vi "3_AdvancedDemo_MHT3.vi"() -> ()   [LabVIEW 2020]
uses:
  Types/MH_UIThread_Cmds.ctl
  _lib/PQ/MultiHarp/MH_InitInfo.ctl
  Types/MH_UIThread_Data.ctl
  Types/MH_InputChannel.ctl
  _lib/PQ/MultiHarp/MH_RefSource.ctl
  _lib/PQ/MultiHarp/mhlib_x86_x64_UIThread.llb/MH_DllPath_global.vi
  <vilib>/Utility/error.llb/DialogType.ctl
  <vilib>/ErrorRing/Error Ring.xnode
  <vilib>/Utility/error.llb/Error Cluster From Error Code.vi
  Types/MH_DataProcThread_QCmds.ctl
  Types/MH_DataProcThread_QData.ctl
  Types/MH_VisThread_QCmds.ctl
  Types/MH_VisThread_QData.ctl
  Types/MH_VisThread_Data.ctl
  _lib/PQ/MultiHarp/MH_LibVersion_global.vi
  _lib/PQ/MultiHarp/MH_MeasMode.ctl
  Types/MH_SetInpChanData.ctl
  Types/MH_SetInpChanCmds.ctl
panel:
  in  "Settings":bool=TRUE
  in  "Run continuously":bool caption="Conti."
  in  "Start":bool
  in  "Scale":bool
  out "CountRates":i32[](graph)
  in  "AllChannels":T1={"Enable"=TRUE, "Offset"=0, "Level"=-100, "Edge"=0, "DeadTime"=1000, "UseDeadTime"=FALSE, "SetEnableAllChan"=TRUE, "SetEdgeAllChan"=TRUE, "SetLevelAllChan"=TRUE, "SetOffsetAllChan"=TRUE, "SetUseDTAllChan"=TRUE, "SetDeadTAllChan"=TRUE} {"DeadTime" min=800 max=160000 step=1; "Edge" items=["falling", "rising"]; "Offset" min=-100000 max=100000 step=10; "Level" min=-1200 max=1200 step=1}
  in  "HistoAcqTime":dbl=1.0 caption="Hist.Int.Time  s" min=0.1 max=360000.0 step=0.1
  in  "AcqTime":i32=360000000 caption="T3Acqu.       ms" min=1 max=360000 step=1
  in  "Binning":i32(ring) caption="Resol.            ps" items=["10", "20", "40", "80", "160", "320", "640", "1280", "2560", "5120", "10240", "20480", "40960", "81920", "163840", "327680", "655360", "1310720", "2621440", "5242880", "10485760", "20971520", "41943040"]
  in  "HistoOffset":i32 caption="Offset            ns" min=0 max=100000000 step=1
  out "DeltaT":dbl=6.553665536655367 caption="T.Tr.Resol.   ms" format="%.2f"
  in  "BitShift":i32=15 min=0 max=32 step=1
  in  "OvlLevel":u32=4294967295 caption="Ovl.Level" min=1024 max=65536 step=1024
  in  "StopOvl.":bool=TRUE
  out "TTraceGraph":T2(graph)={49.38852226226715, "Resolution"=0.00655367864414373, "Histogram"=[]}
  out "HistoGraph":cluster{dbl, "Resol":dbl, "Histos":u32[][]}(graph)={0.0, "Resol"=0.08, "Histos"=[]}
  in  "SyncDeadTime":i32=1000 caption="Dead T.   ps" min=800 max=160000 step=1
  in  "UseDeadTime":bool caption="Use DT."
  in  "SyncEdge":i32(ring) caption="Edge" items=["falling", "rising"]
  in  "SyncDivider":i32(ring) caption="Divider" items=["1", "2", "4", "8", "16"]
  in  "SyncOffset":i32 caption="Offset      ps" min=-100000 max=100000 step=10
  in  "SyncLevel":i32=-100 caption="Level      mV" min=-1200 max=1200 step=1
  in  "Channels":T3[](array[typedef])=[{"Name"="Inp.Chan 1", "Enable"=TRUE, "Edge"=0, "Level"=-100, "Offset"=0, "UseDeadTime"=FALSE, "DeadTime"=1000}, {"Name"="Inp.Chan 2", "Enable"=TRUE, "Edge"=0, "Level"=-100, "Offset"=0, "UseDeadTime"=FALSE, "DeadTime"=1000}, {"Name"="Inp.Chan 3", "Enable"=TRUE, "Edge"=0, "Level"=-100, "Offset"=0, "UseDeadTime"=FALSE, "DeadTime"=1000}, {"Name"="Inp.Chan 4", "Enable"=TRUE, "Edge"=0, "Level"=-100, "Offset"=0, "UseDeadTime"=FALSE, "DeadTime"=1000}, {"Name"="Inp.Chan 5", "Enable"=TRUE, "Edge"=0, "Level"=-100, "Offset"=0, "UseDeadTime"=FALSE, "DeadTime"=1000}, {"Name"="Inp.Chan 6", "Enable"=TRUE, "Edge"=0, "Level"=-100, "Offset"=0, "UseDeadTime"=FALSE, "DeadTime"=1000}, {"Name"="Inp.Chan 7", "Enable"=TRUE, "Edge"=0, "Level"=-100, "Offset"=0, "UseDeadTime"=FALSE, "DeadTime"=1000}, {"Name"="Inp.Chan 8", "Enable"=TRUE, "Edge"=0, "Level"=-100, "Offset"=0, "UseDeadTime"=FALSE, "DeadTime"=1000}, {"Name"="Inp.Chan 9", "Enable"=TRUE, "Edge"=0, "Level"=-100, "Offset"=0, "UseDeadTime"=FALSE, "DeadTime"=1000}, {"Name"="Inp.Chan 10", "Enable"=TRUE, "Edge"=0, "Level"=-100, "Offset"=0, "UseDeadTime"=FALSE, "DeadTime"=1000}, {"Name"="Inp.Chan 11", "Enable"=TRUE, "Edge"=0, "Level"=-100, "Offset"=0, "UseDeadTime"=FALSE, "DeadTime"=1000}, {"Name"="Inp.Chan 12", "Enable"=TRUE, "Edge"=0, "Level"=-100, "Offset"=0, "UseDeadTime"=FALSE, "DeadTime"=1000}, {"Name"="Inp.Chan 13", "Enable"=TRUE, "Edge"=0, "Level"=-100, "Offset"=0, "UseDeadTime"=FALSE, "DeadTime"=1000}, {"Name"="Inp.Chan 14", "Enable"=TRUE, "Edge"=0, "Level"=-100, "Offset"=0, "UseDeadTime"=FALSE, "DeadTime"=1000}, {"Name"="Inp.Chan 15", "Enable"=TRUE, "Edge"=0, "Level"=-100, "Offset"=0, "UseDeadTime"=FALSE, "DeadTime"=1000}, {"Name"="Inp.Chan 16", "Enable"=TRUE, "Edge"=0, "Level"=-100, "Offset"=0, "UseDeadTime"=FALSE, "DeadTime"=1000}] {"DeadTime" min=800 max=160000 step=1; "Edge" items=["falling", "rising"]; "Offset" min=-100000 max=100000 step=10; "Level" min=-1200 max=1200 step=1}
  out "SyncRate":string="Sync Rate: 4999940 cps\n"
  out "OverRun":bool caption="Overrun:"
  out "Status":string="Elements in Q: 0"
  # "All Channels"
  # "Acquisition"
  # "Sync"
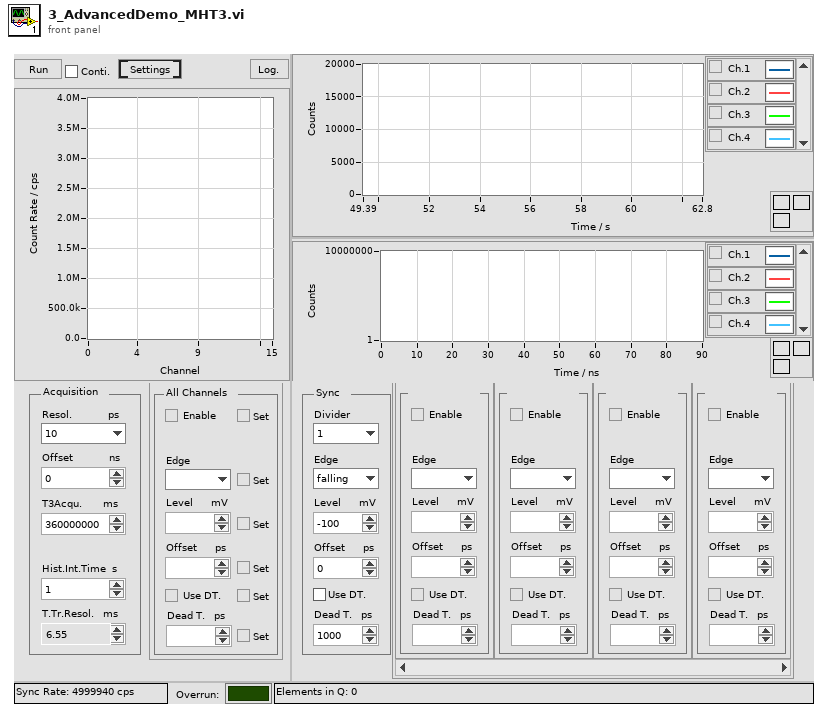
[diagram p1: front panel]
types:
  T1 = cluster{"Enable":bool, "Offset":i32, "Level":i32, "Edge":i32, "DeadTime":i32, "UseDeadTime":bool, "SetEnableAllChan":bool, "SetEdgeAllChan":bool, "SetLevelAllChan":bool, "SetOffsetAllChan":bool, "SetUseDTAllChan":bool, "SetDeadTAllChan":bool}
  T2 = cluster{dbl, "Resolution":dbl, "Histogram":u32[][]}
  T3 = typedef "MH_InputChannel.ctl" = cluster{"Name":string, "Enable":bool, "Edge":i32, "Level":i32, "Offset":i32, "UseDeadTime":bool, "DeadTime":i32}
  T4 = typedef "MH_DataProcThread_QCmds.ctl" = enum16{"Exit", "Proc", "Init", "SetShift", "SetNumChannels", "SetHistAcqTime"}
  T5 = typedef "MH_VisThread_Data.ctl" = cluster{"Resol":dbl, "DeltaT":dbl, "NumChannels":i32}
  T6 = typedef "MH_VisThread_QData.ctl" = cluster{"Histos":u32[][], "Cmd":T7, "TimeTrace":u32[][], "Bin":i32, "Total bin":u64, "Status":string, "Resol":dbl, "DeltaT":dbl, "nChannels":i32}
  T7 = typedef "MH_VisThread_QCmds.ctl" = enum16{"_none_", "Resol", "nChannels", "DeltaT", "Histo", "TTrace", "Status"}
  T8 = typedef "MH_DataProcThread_QData.ctl" = cluster{"Cmd":T4, "nActual":i32, "Buffer":u32[], "TickCount":u32, "Param":i32}
  T9 = typedef "MH_UIThread_Data.ctl" = cluster{"Init Info":T10, "DevIdx":i32, "SyncDivider":i32, "SyncOffset":i32, "SyncLevel":i32, "Channels":T3[], "CurrentChannels":i32[], "AcqTime":i32, "Binning":i32, "HistoOffset":i32, "HistoLen":i32, "StopOvl.":bool, "OvlLevel":u32, "SyncEdge":i32, "StartMeas":bool, "HistoLength":i32, "Resolution":dbl, "Run cont.":bool, "Status":string, "SyncRate":i32, "BitShift":i32, "HistoAcqTime":dbl, "SyncRateStart":i32, "UseDeadTime":bool, "SyncDeadTime":i32, "SetInpChan":T11[]}
  T10 = typedef "MH_InitInfo.ctl" = cluster{"Library Version":string, "Serial No.":string, "Model":string, "Partnum":string, "Version":string, "features":i32, "nchannels":i32, "Base Resolution":dbl, "Bin Steps":i32}
  T11 = typedef "MH_SetInpChanData.ctl" = cluster{"Channel":i32, "Cmds":T12[], "Changed":cluster{"Name":bool, "Enable":bool, "Edge":bool, "Level":bool, "Offset":bool, "UseDeadTime":bool, "DeadTime":bool}}
  T12 = typedef "MH_SetInpChanCmds.ctl" = enum16{"SetInpChanEnable", "SetInpChanOffset", "SetInpChanDeadTime", "SetInpChanTrg"}
  T13 = typedef "MH_UIThread_Cmds.ctl" = enum16{"Idle", "Init", "SetInpChan", "SetSyncDivider", "SetSyncTrg", "SetSyncOffset", "SetSyncDeadTime", "SetBinning", "SetHistoOffset", "SetHistoLen", "SetStopOvl", "SetBitShift", "SetHistoAcqTime", "GetRates", "GetAllRates", "StartMeas", "StopMeas", "AbortMeas", "GetResolution", "GetHistos", "GetAllHistos", "ReadFiFo", "WriteStatus", "Resize", "EnableControls", "DisableControls", "Error", "Exit"}
  T14 = enum8{"Enabled", "Disabled", "Disabled and Grayed Out"}
  T15 = cluster{"[0]":bool, "[1]":bool, "[2]":bool, "[3]":bool, "[4]":bool, "[5]":bool}
  T16 = typedef "MH_MeasMode.ctl" = i32
  T17 = typedef "MH_RefSource.ctl" = enum16{"INTERNAL", "EXTERNAL_10MHZ", "WR_MASTER_GENERIC", "WR_SLAVE_GENERIC", "WR_GRANDM_GENERIC", "EXTN_GPS_PPS", "EXTN_GPS_PPS_UART", "WR_MASTER_MHARP", "WR_SLAVE_MHARP", "WR_GRANDM_MHARP"}
  T18 = typedef "DialogType.ctl" = u16
  T19 = cluster{"T0":dbl, "dt":dbl, "TimeTrace_out":u32[][]}
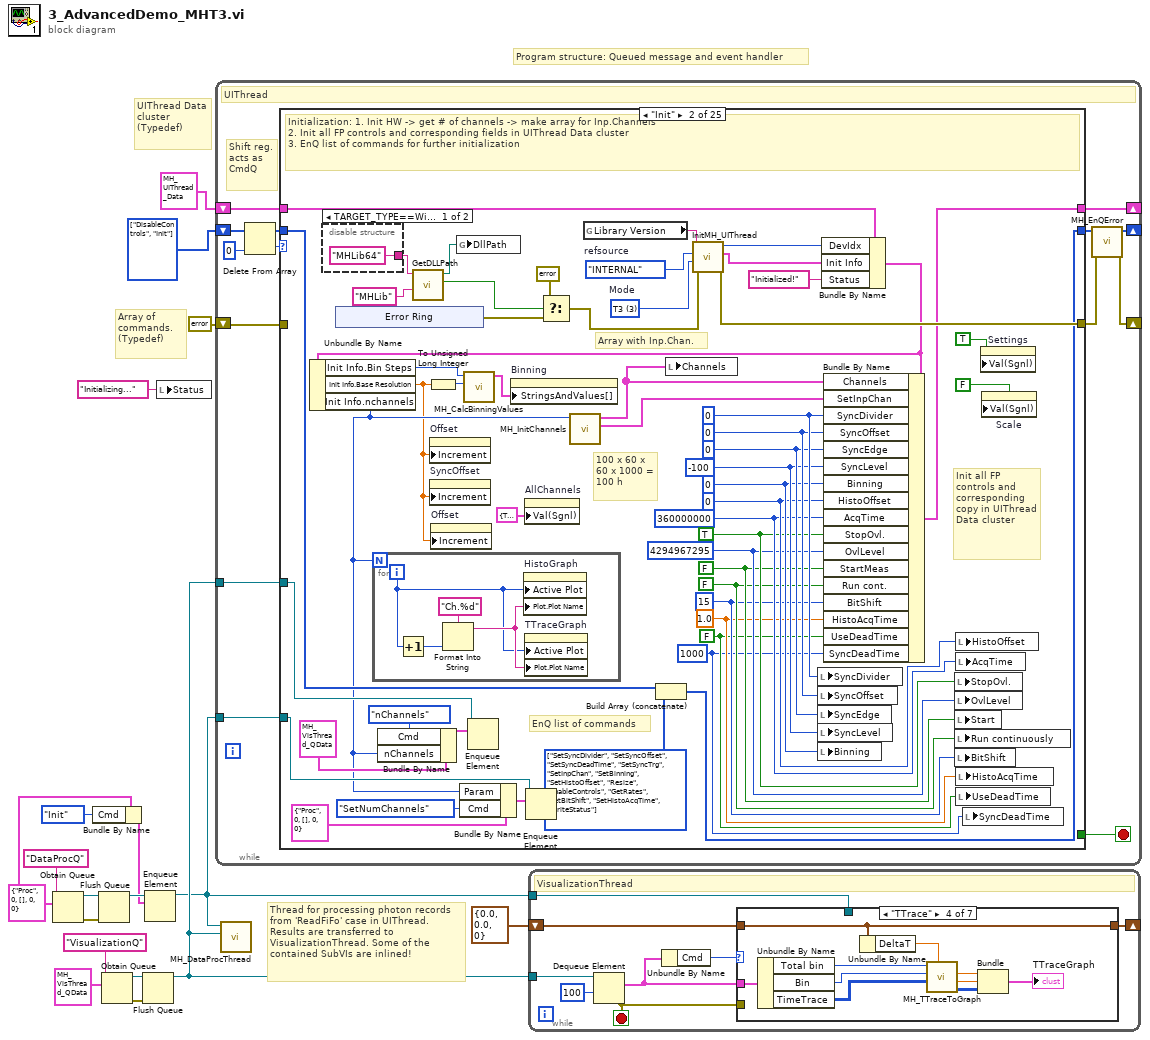
[diagram p0: block diagram]
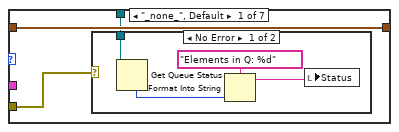
[diagram p2: hidden frame]
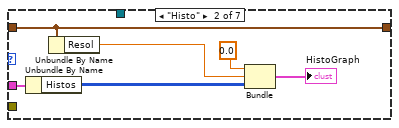
[diagram p4: hidden frame]
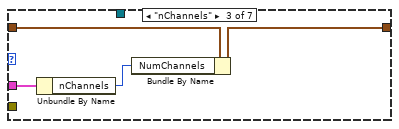
[diagram p5: hidden frame]
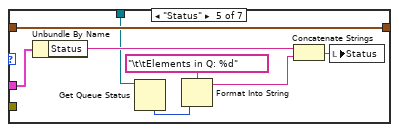
[diagram p6: hidden frame]
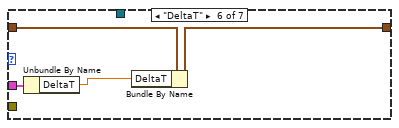
[diagram p7: hidden frame]
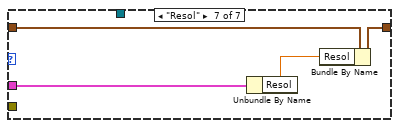
[diagram p8: hidden frame]
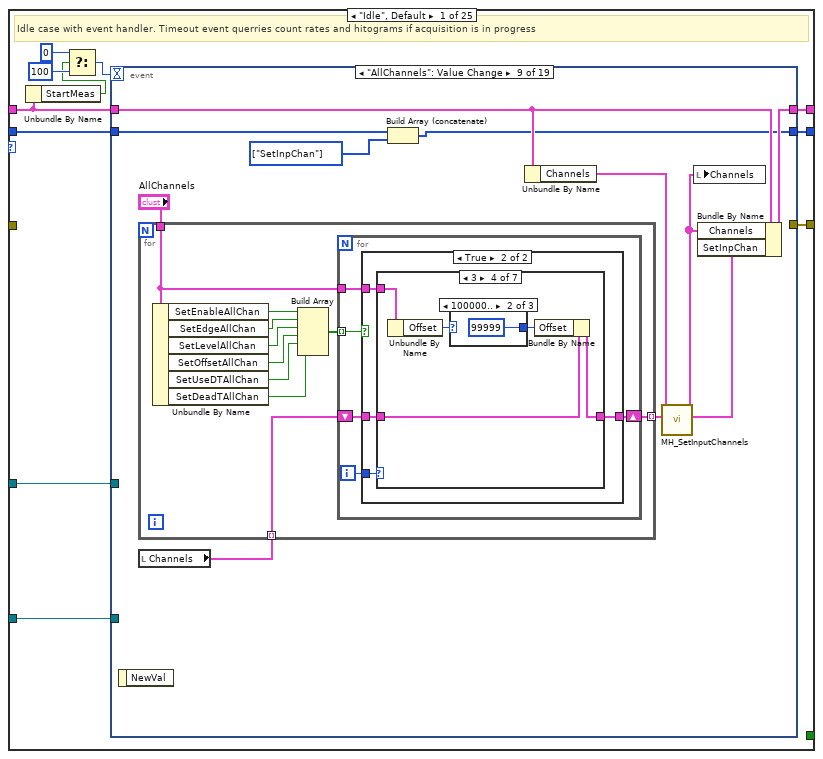
[diagram p9: hidden frame]
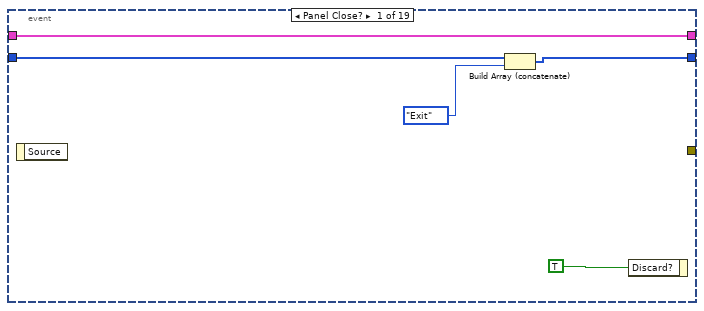
[diagram p10: hidden frame]
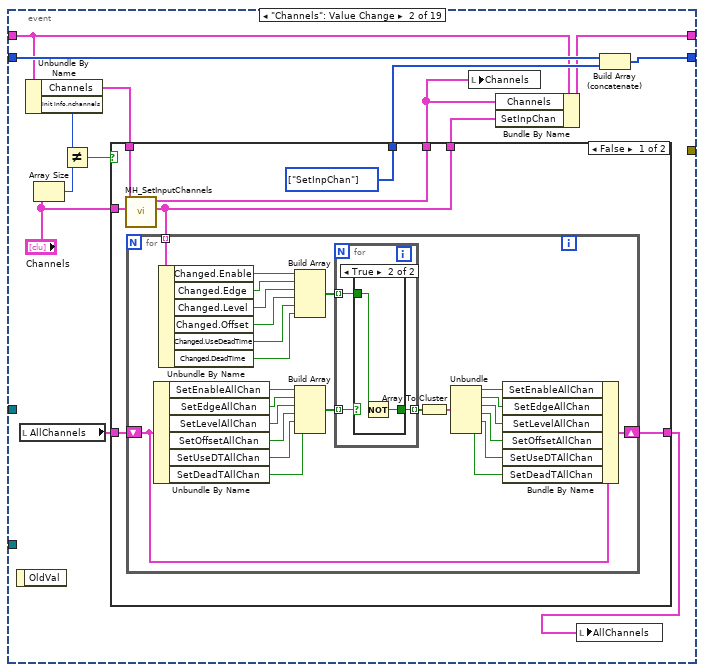
[diagram p11: hidden frame]
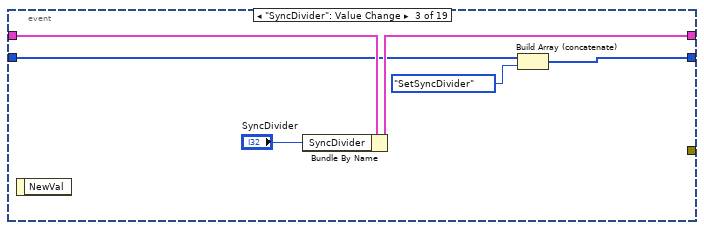
[diagram p14: hidden frame]
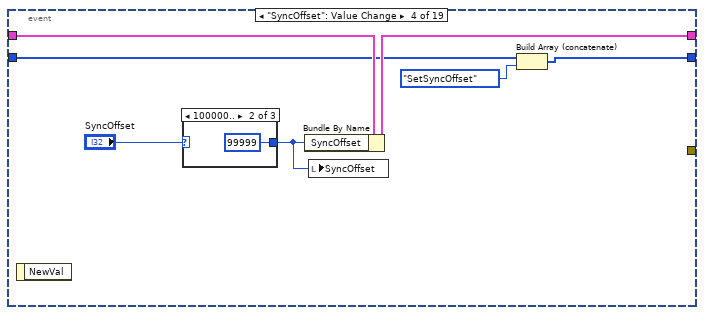
[diagram p15: hidden frame]
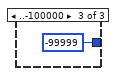
[diagram p17: hidden frame]
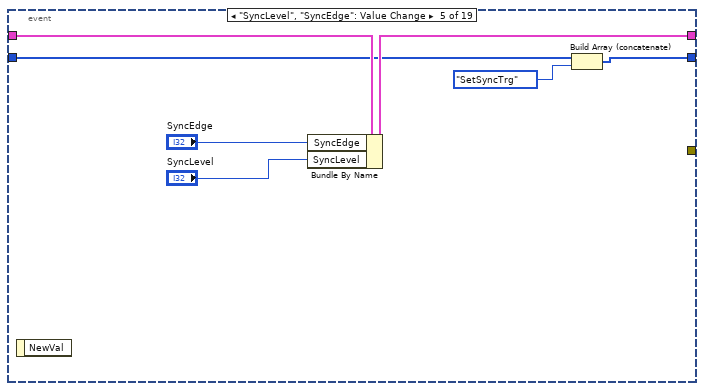
[diagram p18: hidden frame]
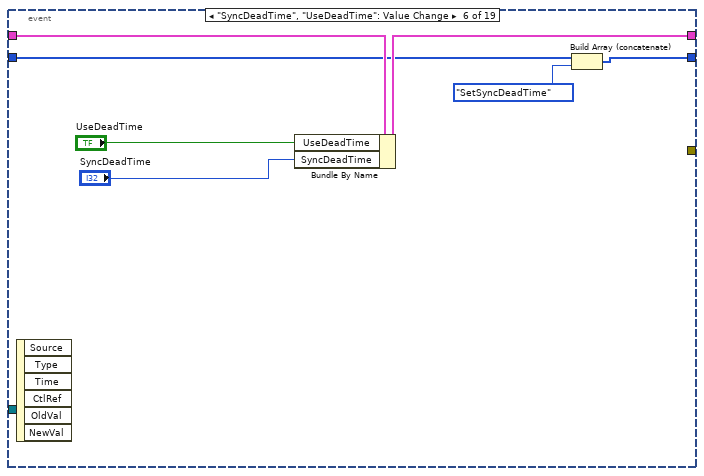
[diagram p19: hidden frame]
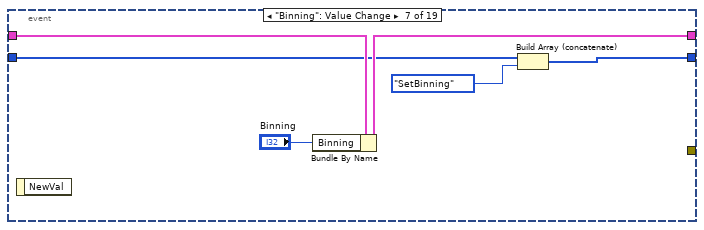
[diagram p20: hidden frame]
diagram:
  w4 = T8 {"Cmd"=enum."Proc", "nActual"=0, "Buffer"=[], "TickCount"=0, "Param"=0} ("MH_DataProcThread_QData")
  w17 = T13[] [enum."DisableControls", enum."Init"] items=["Idle", "Init", "SetInpChan", "SetSyncDivider", "SetSyncTrg", "SetSyncOffset", "SetSyncDeadTime", "SetBinning", "SetHistoOffset", "SetHistoLen", "SetStopOvl", "SetBitShift", "SetHistoAcqTime", "GetRates", "GetAllRates", "StartMeas", "StopMeas", "AbortMeas", "GetResolution", "GetHistos", "GetAllHistos", "ReadFiFo", "WriteStatus", "Resize", "EnableControls", "DisableControls", "Error", "Exit"]
  # "Thread for processing photon records from 'ReadFiFo' case in UIThread. Results are transferred to VisualizationThread. Some of the contained SubVIs are inlined!"
  # "Array of commands.\n(Typedef)"
  # "Program structure: Queued message and event handler"
  # "UIThread Data cluster\n(Typedef)"
  n1 = Obtain Queue(name (unnamed)="DataProcQ", element data type=w4) -> (queue out=w14:refnum<queue>, error out=w13:errorcluster)  [unwired: 3 in, 1 out]
  n2 = Bundle By Name(cluster=w4, "Cmd"=MH_DataProcThread_QCmds."Init") -> (w2:T8)
  n3 = Flush Queue(queue=w14, error in (no error)=w13) -> (queue out=w5:refnum<queue>)  [unwired: 2 out]
  n4 = Obtain Queue(name (unnamed)="VisualizationQ", element data type=T6 {"Histos"=[], "Cmd"=enum."_none_", "TimeTrace"=[], "Bin"=0, "Total bin"=0, "Status"="", "Resol"=0.0, "DeltaT"=0.0, "nChannels"=0} ("MH_GUIThread_QData")) -> (queue out=w12:refnum<queue>, error out=w11:errorcluster)  [unwired: 3 in, 1 out]
  n5 = Flush Queue(queue=w12, error in (no error)=w11) -> (queue out=w7:refnum<queue>)  [unwired: 2 out]
  n6 = Enqueue Element(queue=w5, element=w2) -> (queue out=w1:refnum<queue>)  [unwired: 2 in, 2 out]
  n7 = local write "Status"("Initializing..." ("Status")) -> ()
  n8 = while {
    shift-right: [w21] -> _
    shift-left: w17 -> [w28]
    shift-right: [w31] -> _
    shift-left: T9 {"Init Info"={"Library Version"="", "Serial No."="", "Model"="", "Partnum"="", "Version"="", "features"=0, "nchannels"=0, "Base Resolution"=0.0, "Bin Steps"=0}, "DevIdx"=0, "SyncDivider"=1, "SyncOffset"=0, "SyncLevel"=50, "Channels"=[], "CurrentChannels"=[], "AcqTime"=1, "Binning"=1, "HistoOffset"=1, "HistoLen"=1024, "StopOvl."=FALSE, "OvlLevel"=1024, "SyncEdge"=10, "StartMeas"=FALSE, "HistoLength"=0, "Resolution"=0.0, "Run cont."=FALSE, "Status"="", "SyncRate"=0, "BitShift"=0, "HistoAcqTime"=0.0, "SyncRateStart"=0, "UseDeadTime"=FALSE, "SyncDeadTime"=800, "SetInpChan"=[]} -> [w30]
    shift-right: [w23] -> _
    shift-left: errorcluster {"status"=FALSE, "code"=0, "source"=""} ("error IO") -> [w29]
    tunnel: w1 -> [w20]
    tunnel: w7 -> [w19]
    stop <- w32 stop-if-true
    # "Shift reg.\nacts as\nCmdQ"
    # "UIThread"
    n9 = Delete From Array(array=w28, index=0) -> (deleted portion=w26:T13, array with subset deleted=w25:T13[])  [unwired: 1 in]
    n10 = case shown="\"Init\"" w26 {
      tunnel: [w43 w355 w378 w440 w449 w461 w467 w474 w482 w489 w509 w521 w524 w596 w619 w624 w637 w654 w655 w681 w694 w701 w713 w719 w725] -> w22
      tunnel: [_ _ _ _ _ _ _ _ _ _ _ _ _ _ _ _ _ _ _ _ _ _ _ _ TRUE] -> w32
      tunnel: [w42 w336 w379 w442 w450 w462 w471 w478 w483 w490 w494 w511 w533 w588 w611 w627 w639 w650 w665 w680 w682 w700 w712 w720 w728] -> w31
      tunnel: w30 -> [w39 w341 w379 w442 w450 w462 w471 w478 w483 w490 w494 w511 w523 w589 w612 w628 w640 w651 w665 w680 w682 w700 w712 w720 w728]
      tunnel: [w40 w358 w373 w438 w448 w460 w470 w477 w481 w488 _ _ w529 w595 w622 w630 w642 w652 w660 _ _ _ _ _ w726] -> w24
      tunnel: w29 -> [_ _ _ _ _ _ _ _ _ _ _ _ _ _ _ _ _ _ _ _ _ _ _ w721 _]
      tunnel: w25 -> [w41 w357 w378 w440 w449 w461 w467 w473 w482 w489 w509 w521 w525 w596 w620 w625 w637 w654 w656 w681 w694 w701 w713 _ w725]
      tunnel: w20 -> [w34 w334 _ _ _ _ _ _ _ _ w495 w512 _ _ w616 _ _ _ w657 _ _ _ _ _ w724]
      tunnel: w19 -> [w33 w327 _ _ _ _ _ _ _ _ w496 _ _ _ _ _ _ w647 _ _ _ _ _ _ w723]
      frame "Idle", Default {
        # "Idle case with event handler. Timeout event querries count rates and hitograms if acquisition is in progress"
        n11 = Unbundle By Name(w39) -> ("StartMeas"=w37:bool)
        n12 = Select(t=0, s=w37, f=100) -> (s? t:f=w36:i32)
        n13 = event shown="[8] \"AllChannels\": Value Change" {
          selector: _ -> [_ _ _ _ _ _ _ _ _ _ _ _ _ _ _ _ _ _ _]
          dyn-events: _ -> [_ _ _ _ _ _ _ _ _ _ _ _ _ _ _ _ _ _ _]
          timeout: w36 -> [_ _ _ _ _ _ _ _ _ _ _ _ _ _ _ _ _ _ _]
          tunnel: [w44 w61 w103 w111 w120 w128 w134 w140 w145 w205 w210 w217 w232 w250 w262 w280 w286 w294 w304] -> w43
          tunnel: [w47 w53 w107 w114 w124 w131 w137 w143 w150 w207 w213 w220 w231 w254 w261 w278 w285 w293 w307] -> w42
          tunnel: w39 -> [w47 w54 w108 w115 w125 w132 w138 w144 w151 w208 w214 w221 w231 w255 w259 w279 w285 w293 w307]
          tunnel: w41 -> [w46 w62 w105 w113 w122 w130 w136 w142 w146 w205 w211 w219 w233 w251 w263 w280 w286 w294 w305]
          tunnel: [_ _ _ _ _ _ _ _ _ _ _ _ w227 _ _ _ _ _ _] -> w40
          tunnel: w34 -> [_ _ _ _ _ _ _ _ _ _ _ _ _ _ _ _ _ _ _]
          tunnel: w33 -> [_ _ _ _ _ _ _ _ _ _ _ _ _ _ _ _ _ _ _]
          event Panel Close? {
            n14 = event-data() -> ()  [unwired: 1 in, 1 out]
            n15 = Build Array (concatenate)(w46, MH_UIThread_Cmds."Exit") -> (w44:T13[])
            n16 = event-data("Discard?"=TRUE) -> ()  [unwired: 1 in, 1 out]
          }
          event "Channels": Value Change {
            n17 = event-data() -> ()  [unwired: 1 in, 1 out]
            n18 = local read "AllChannels"() -> (w49:T1)
            n19 = Unbundle By Name(w54) -> ("Channels"=w56:T3[], "Init Info.nchannels"=w58:i32)
            n20 = Array Size(array="Channels") -> (size(s)=w59:i32)
            n21 = Not Equal?(x=w58, y=w59) -> (x != y?=w57:bool)
            n22 = case shown="False" w57 {
              tunnel: "Channels" -> [w68 _]
              tunnel: [w67 w102] -> w51
              tunnel: w56 -> [w69 w102]
              tunnel: [w65 _] -> w52
              tunnel: [w66 _] -> w55
              tunnel: w49 -> [w64 w101]
              tunnel: [w63 w101] -> w50
              frame False {
                w66 = T13[] [enum."SetInpChan"] items=["Idle", "Init", "SetInpChan", "SetSyncDivider", "SetSyncTrg", "SetSyncOffset", "SetSyncDeadTime", "SetBinning", "SetHistoOffset", "SetHistoLen", "SetStopOvl", "SetBitShift", "SetHistoAcqTime", "GetRates", "GetAllRates", "StartMeas", "StopMeas", "AbortMeas", "GetResolution", "GetHistos", "GetAllHistos", "ReadFiFo", "WriteStatus", "Resize", "EnableControls", "DisableControls", "Error", "Exit"] ("array")
                n23 = call "MH_SetInputChannels.vi"("Channels new"=w68, "Channels old"=w69) -> ("SetInpChan"=w65:T11[], "Channels"=w67:T3[])  [unwired: 8 in]
                n24 = for {
                  tunnel: w65 -> [w94] mode=indexing
                  shift-right: [w76] -> w63
                  shift-left: w64 -> [w78]
                  n25 = Unbundle By Name(w78) -> ("SetEnableAllChan"=w87:bool, "SetEdgeAllChan"=w86:bool, "SetLevelAllChan"=w85:bool, "SetOffsetAllChan"=w84:bool, "SetUseDTAllChan"=w83:bool, "SetDeadTAllChan"=w82:bool)
                  n26 = Unbundle By Name(w94) -> ("Changed.Enable"=w93:bool, "Changed.Edge"=w92:bool, "Changed.Level"=w91:bool, "Changed.Offset"=w90:bool, "Changed.UseDeadTime"=w89:bool, "Changed.DeadTime"=w88:bool)
                  n27 = Build Array(w93, w92, w91, w90, w89, w88) -> (w80:bool[])
                  n28 = Build Array(w87, w86, w85, w84, w83, w82) -> (w81:bool[])
                  n29 = for {
                    tunnel: w81 -> [w97] mode=indexing
                    tunnel: w80 -> [w95] mode=indexing
                    tunnel: [w96] -> w79 mode=indexing
                    n30 = case shown="True" w97 {
                      selector: w97 -> [w98 _]
                      tunnel: [w98 w99] -> w96
                      tunnel: w95 -> [_ w100]
                      frame False {
                      }
                      frame True {
                        n31 = Not(x=w100) -> (.not. x?=w99:bool)
                      }
                    }
                  }
                  n32 = Array To Cluster(array=w79) -> (cluster=w77:T15)
                  n33 = Unbundle(w77) -> ("[0]"=w75:bool, "[1]"=w74:bool, "[2]"=w73:bool, "[3]"=w72:bool, "[4]"=w71:bool, "[5]"=w70:bool)
                  n34 = Bundle By Name(cluster=w78, "SetEnableAllChan"=w75, "SetEdgeAllChan"=w74, "SetLevelAllChan"=w73, "SetOffsetAllChan"=w72, "SetUseDTAllChan"=w71, "SetDeadTAllChan"=w70) -> (w76:T1)
                }
              }
              frame True {
              }
            }
            n35 = local write "Channels"(w51) -> ()
            n36 = Bundle By Name(cluster=w54, "Channels"=w51, "SetInpChan"=w52) -> (w53:T9)
            n37 = local write "AllChannels"(w50) -> ()
            n38 = Build Array (concatenate)(w62, w55) -> (w61:T13[])
          }
          event "SyncDivider": Value Change {
            n39 = event-data() -> ()  [unwired: 1 in, 1 out]
            n40 = Bundle By Name(cluster=w108, "SyncDivider"="SyncDivider") -> (w107:T9)
            n41 = Build Array (concatenate)(w105, MH_UIThread_Cmds."SetSyncDivider") -> (w103:T13[])
          }
          event "SyncOffset": Value Change {
            n42 = event-data() -> ()  [unwired: 1 in, 1 out]
            n43 = case shown="100000.." "SyncOffset" {
              selector: "SyncOffset" -> [w116 _ _]
              tunnel: [w116 99999 ("SyncOffset") -99999 ("SyncOffset")] -> w109
              frame Default {
              }
              frame 100000.. {
              }
              frame ..-100000 {
              }
            }
            n44 = Bundle By Name(cluster=w115, "SyncOffset"=w109) -> (w114:T9)
            n45 = local write "SyncOffset"(w109) -> ()
            n46 = Build Array (concatenate)(w113, MH_UIThread_Cmds."SetSyncOffset") -> (w111:T13[])
          }
          event "SyncLevel", "SyncEdge": Value Change {
            n47 = event-data() -> ()  [unwired: 1 in, 1 out]
            n48 = Bundle By Name(cluster=w125, "SyncEdge"="SyncEdge", "SyncLevel"="SyncLevel") -> (w124:T9)
            n49 = Build Array (concatenate)(w122, MH_UIThread_Cmds."SetSyncTrg") -> (w120:T13[])
          }
          event "SyncDeadTime", "UseDeadTime": Value Change {
            n50 = event-data() -> ()  [unwired: 1 in, 6 out]
            n51 = Bundle By Name(cluster=w132, "UseDeadTime"="UseDeadTime", "SyncDeadTime"="SyncDeadTime") -> (w131:T9)
            n52 = Build Array (concatenate)(w130, MH_UIThread_Cmds."SetSyncDeadTime") -> (w128:T13[])
          }
          event "Binning": Value Change {
            n53 = event-data() -> ()  [unwired: 1 in, 1 out]
            n54 = Bundle By Name(cluster=w138, "Binning"="Binning") -> (w137:T9)
            n55 = Build Array (concatenate)(w136, MH_UIThread_Cmds."SetBinning") -> (w134:T13[])
          }
          event "HistoOffset": Value Change {
            n56 = event-data() -> ()  [unwired: 1 in, 1 out]
            n57 = Bundle By Name(cluster=w144, "HistoOffset"="HistoOffset") -> (w143:T9)
            n58 = Build Array (concatenate)(w142, MH_UIThread_Cmds."SetHistoOffset") -> (w140:T13[])
          }
          event "AllChannels": Value Change {
            w147 = T13[] [enum."SetInpChan"] items=["Idle", "Init", "SetInpChan", "SetSyncDivider", "SetSyncTrg", "SetSyncOffset", "SetSyncDeadTime", "SetBinning", "SetHistoOffset", "SetHistoLen", "SetStopOvl", "SetBitShift", "SetHistoAcqTime", "GetRates", "GetAllRates", "StartMeas", "StopMeas", "AbortMeas", "GetResolution", "GetHistos", "GetAllHistos", "ReadFiFo", "WriteStatus", "Resize", "EnableControls", "DisableControls", "Error", "Exit"] ("array")
            n59 = event-data() -> ()  [unwired: 1 in, 1 out]
            n60 = local read "Channels"() -> (w154:T3[])
            n61 = for {
              tunnel: w154 -> [w158] mode=indexing
              tunnel: "AllChannels" -> [w157]
              tunnel: [w156] -> w153 mode=indexing
              n62 = Unbundle By Name(w157) -> ("SetEnableAllChan"=w159:bool, "SetEdgeAllChan"=w160:bool, "SetLevelAllChan"=w161:bool, "SetOffsetAllChan"=w162:bool, "SetUseDTAllChan"=w163:bool, "SetDeadTAllChan"=w164:bool)
              n63 = Build Array(w159, w160, w161, w162, w163, w164) -> (w165:bool[])
              n64 = for {
                tunnel: w165 -> [w170] mode=indexing
                shift-right: [w167] -> w156
                shift-left: w158 -> [w168]
                tunnel: w157 -> [w166]
                i -> [w169]
                n65 = case shown="True" w170 {
                  tunnel: w169 -> [_ w175]
                  tunnel: w166 -> [_ w174]
                  tunnel: w168 -> [w171 w173]
                  tunnel: [w171 w172] -> w167
                  frame False {
                  }
                  frame True {
                    n66 = case shown="3" w175 {
                      tunnel: w174 -> [w179 w183 w187 w192 w199 w203 _]
                      tunnel: w173 -> [w178 w182 w186 w191 w198 w202 w204]
                      tunnel: [w176 w180 w184 w190 w196 w200 w204] -> w172
                      frame 0 {
                        n67 = Unbundle By Name(w179) -> ("Enable"=w177:bool)
                        n68 = Bundle By Name(cluster=w178, "Enable"=w177) -> (w176:T3)
                      }
                      frame 1 {
                        n69 = Unbundle By Name(w183) -> ("Edge"=w181:i32)
                        n70 = Bundle By Name(cluster=w182, "Edge"=w181) -> (w180:T3)
                      }
                      frame 2 {
                        n71 = Unbundle By Name(w187) -> ("Level"=w185:i32)
                        n72 = Bundle By Name(cluster=w186, "Level"=w185) -> (w184:T3)
                      }
                      frame 3 {
                        n73 = Unbundle By Name(w192) -> ("Offset"=w189:i32)
                        n74 = case shown="100000.." w189 {
                          selector: w189 -> [w193 _ _]
                          tunnel: [w193 99999 ("SyncOffset") -99999 ("SyncOffset")] -> w188
                          frame Default {
                          }
                          frame 100000.. {
                          }
                          frame ..-100000 {
                          }
                        }
                        n75 = Bundle By Name(cluster=w191, "Offset"=w188) -> (w190:T3)
                      }
                      frame 4 {
                        n76 = Unbundle By Name(w199) -> ("UseDeadTime"=w197:bool)
                        n77 = Bundle By Name(cluster=w198, "UseDeadTime"=w197) -> (w196:T3)
                      }
                      frame 5 {
                        n78 = Unbundle By Name(w203) -> ("DeadTime"=w201:i32)
                        n79 = Bundle By Name(cluster=w202, "DeadTime"=w201) -> (w200:T3)
                      }
                      frame Default {
                      }
                    }
                  }
                }
              }
            }
            n80 = Build Array (concatenate)(w146, w147) -> (w145:T13[])
            n81 = Unbundle By Name(w151) -> ("Channels"=w152:T3[])
            n82 = call "MH_SetInputChannels.vi"("Channels new"=w153, "Channels old"=w152) -> ("SetInpChan"=w148:T11[], "Channels"=w149:T3[])  [unwired: 8 in]
            n83 = local write "Channels"(w149) -> ()
            n84 = Bundle By Name(cluster=w151, "Channels"=w149, "SetInpChan"=w148) -> (w150:T9)
          }
          event "AcqTime": Value Change {
            n85 = event-data() -> ()  [unwired: 1 in, 1 out]
            n86 = Bundle By Name(cluster=w208, "AcqTime"="AcqTime") -> (w207:T9)
          }
          event "HistoAcqTime": Value Change {
            n87 = event-data() -> ()  [unwired: 1 in, 1 out]
            n88 = Bundle By Name(cluster=w214, "HistoAcqTime"="HistoAcqTime") -> (w213:T9)
            n89 = Build Array (concatenate)(w211, MH_UIThread_Cmds."SetHistoAcqTime") -> (w210:T13[])
          }
          event "OvlLevel", "StopOvl.": Value Change {
            n90 = event-data() -> ()  [unwired: 1 in, 1 out]
            n91 = Bundle By Name(cluster=w221, "StopOvl."="StopOvl.", "OvlLevel"="OvlLevel") -> (w220:T9)
            n92 = Build Array (concatenate)(w219, MH_UIThread_Cmds."SetStopOvl") -> (w217:T13[])
          }
          event Timeout {
            n93 = event-data() -> ()  [unwired: 1 in, 1 out]
            n94 = Unbundle By Name(w231) -> ("DevIdx"=w229:i32, "StartMeas"=w230:bool, "BitShift"=w226:i32, "SyncRate"=w225:i32)
            n95 = case shown="True" w230 {
              tunnel: w229 -> [_ w249]
              tunnel: [_ w247] -> w228
              tunnel: [_ w244] -> w227
              frame False {
              }
              frame True {
                w245 = T13[] [enum."ReadFiFo"] items=["Idle", "Init", "SetInpChan", "SetSyncDivider", "SetSyncTrg", "SetSyncOffset", "SetSyncDeadTime", "SetBinning", "SetHistoOffset", "SetHistoLen", "SetStopOvl", "SetBitShift", "SetHistoAcqTime", "GetRates", "GetAllRates", "StartMeas", "StopMeas", "AbortMeas", "GetResolution", "GetHistos", "GetAllHistos", "ReadFiFo", "WriteStatus", "Resize", "EnableControls", "DisableControls", "Error", "Exit"]
                w246 = T13[] [enum."StopMeas"] items=["Idle", "Init", "SetInpChan", "SetSyncDivider", "SetSyncTrg", "SetSyncOffset", "SetSyncDeadTime", "SetBinning", "SetHistoOffset", "SetHistoLen", "SetStopOvl", "SetBitShift", "SetHistoAcqTime", "GetRates", "GetAllRates", "StartMeas", "StopMeas", "AbortMeas", "GetResolution", "GetHistos", "GetAllHistos", "ReadFiFo", "WriteStatus", "Resize", "EnableControls", "DisableControls", "Error", "Exit"]
                n96 = call "MH_CTCStatus.vi"("devidx"=w249) -> ("error out"=w244:errorcluster, "ctcstatus"=w248:i32)  [unwired: 8 in, 1 out]
                n97 = Not Equal To 0?(x=w248) -> (x != 0?=w243:bool)
                n98 = Select(t=w246, s=w243, f=w245) -> (s? t:f=w247:T13[])
              }
            }
            n99 = call "CalcRate.vi"("Refresh(ms)"=u32 100) -> ("updated?"=w223:bool)  [unwired: 8 in, 2 out]
            n100 = case shown="True" w223 {
              tunnel: w226 -> [_ w236]
              tunnel: w225 -> [_ w235]
              tunnel: [_ MH_UIThread_Cmds."GetAllRates"] -> w224
              frame False {
              }
              frame True {
                n101 = To Double Precision Float(number=w235) -> (double precision float=w240:dbl)
                n102 = To Double Precision Float(number=w236) -> (double precision float=w241:dbl)
                n103 = Power Of 2(x=w241) -> (2^x=w239:dbl)
                n104 = Multiply(x=w239, y=1000.0) -> (x*y=w238:dbl)
                n105 = Divide(x=w238, y=w240) -> (x/y=w242:dbl)
                n106 = local write "DeltaT"(w242) -> ()
              }
            }
            n107 = Build Array (concatenate)(w233, w228, w224) -> (w232:T13[])
          }
          event "BitShift": Value Change {
            n108 = event-data() -> ()  [unwired: 1 in, 1 out]
            n109 = Bundle By Name(cluster=w255, "BitShift"="BitShift") -> (w254:T9)
            n110 = Build Array (concatenate)(w251, MH_UIThread_Cmds."SetBitShift") -> (w250:T13[])
          }
          event "Start": Value Change {
            n111 = event-data() -> ()  [unwired: 1 in, 1 out]
            n112 = Unbundle By Name(w259) -> ("SyncRate"=w258:i32)
            n113 = Greater Or Equal?(x=w258, y=10) -> (x >= y?=w256:bool)
            n114 = case shown="True" w256 {
              selector: w256 -> [w265 _]
              tunnel: w263 -> [w267 w276]
              tunnel: [w267 w274] -> w262
              tunnel: [w266 w273] -> w261
              tunnel: "Start" -> [_ w272]
              tunnel: w259 -> [w266 w268]
              frame False {
                n115 = local write "Start"(w265) -> ()
                n116 = One Button Dialog(message="SyncRate too low!!!" ("Status")) -> ()  [unwired: 1 in, 1 out]
              }
              frame True {
                w271 = T13[] [enum."SetBitShift", enum."SetHistoAcqTime", enum."StartMeas"] items=["Idle", "Init", "SetInpChan", "SetSyncDivider", "SetSyncTrg", "SetSyncOffset", "SetSyncDeadTime", "SetBinning", "SetHistoOffset", "SetHistoLen", "SetStopOvl", "SetBitShift", "SetHistoAcqTime", "GetRates", "GetAllRates", "StartMeas", "StopMeas", "AbortMeas", "GetResolution", "GetHistos", "GetAllHistos", "ReadFiFo", "WriteStatus", "Resize", "EnableControls", "DisableControls", "Error", "Exit"]
                n117 = Bundle By Name(cluster=w268, "StartMeas"=w272) -> (w273:T9)
                n118 = Build Array(MH_UIThread_Cmds."AbortMeas") -> (w269:T13[])
                n119 = Select(t=w271, s=w272, f=w269) -> (s? t:f=w275:T13[])
                n120 = Build Array (concatenate)(w276, w275) -> (w274:T13[])
              }
            }
          }
          event "Run continuously": Value Change {
            n121 = event-data() -> ()  [unwired: 1 in, 1 out]
            n122 = Bundle By Name(cluster=w279, "Run cont."="Run continuously") -> (w278:T9)
          }
          event "Scale": Value Change {
            n123 = event-data() -> ()  [unwired: 1 in, 1 out]
            n124 = Select(t=u8 0 ("Y Scale.Mapping Mode"), s="Scale", f=u8 1 ("Y Scale.Mapping Mode")) -> (s? t:f=w281:u8)
            n125 = property on="HistoGraph" class="WFGraph (strict)"("YScale.Mapping Mode"=w281) -> ()  [unwired: 2 in, 2 out]
          }
          event "Settings": Value Change {
            n126 = event-data() -> ()  [unwired: 1 in, 1 out]
            n127 = property on="Splitter" class="Splitter"() -> ("Position"=w292:i32)  [unwired: 2 in, 2 out]
            n128 = Select(t=300 ("PosT"), s="Settings", f=0 ("PosF")) -> (s? t:f=w289:i32)
            n129 = Subtract(x=w292, y=w289) -> (x-y=w288:i32)
            n130 = while {
              shift-right: [w303] -> _
              shift-left: w288 -> [w296]
              i -> [w302]
              stop <- w299 stop-if-true
              n131 = property on="Splitter 4" class="Splitter"("Position"=w296) -> (error out=w295:errorcluster)  [unwired: 2 in, 1 out]
              n132 = Greater Or Equal?(x=w302, y=10) -> (x >= y?=w300:bool)
              n133 = Decrement(x=w296) -> (x-1=w303:i32)
              n134 = Unbundle(w295) -> ("status"=w298:bool)  [unwired: 2 out]
              n135 = Not(x=w298) -> (.not. x?=w297:bool)
              n136 = Or(x=w297, y=w300) -> (x .or. y?=w299:bool)
            }
          }
          event Panel Resize {
            n137 = event-data() -> ()  [unwired: 1 in, 1 out]
            n138 = Build Array (concatenate)(w305, MH_UIThread_Cmds."Resize") -> (w304:T13[])
          }
        }
      }
      frame "Init" {
        w314 = 1000 ("SyncDeadTime")
        w315 = FALSE ("UseDeadTime")
        w317 = T16 3 items=["HIST"=0, "T2"=2, "T3"=3]  # Mode
        w319 = MH_RefSource."INTERNAL"  # refsource
        w325 = 1.0 ("HistoAcqTime")
        w326 = 15 ("Value (Signaling)")
        w343 = FALSE ("Run cont.")
        w345 = FALSE ("StartMeas")
        w346 = u32 4294967295 ("OvlLevel")
        w347 = TRUE ("StopOvl.")
        w348 = 360000000 ("AcqTime")
        w349 = 0 ("HistoOffset")
        w350 = 0 ("Binning")
        w351 = -100 ("SyncLevel")
        w352 = 0 ("SyncZeroX")
        w353 = 0 ("SyncOffset")
        w354 = 0 ("SyncDivider")
        w356 = T13[] [enum."SetSyncDivider", enum."SetSyncOffset", enum."SetSyncDeadTime", enum."SetSyncTrg", enum."SetInpChan", enum."SetBinning", enum."SetHistoOffset", enum."Resize", enum."EnableControls", enum."GetRates", enum."SetBitShift", enum."SetHistoAcqTime", enum."WriteStatus"] items=["Idle", "Init", "SetInpChan", "SetSyncDivider", "SetSyncTrg", "SetSyncOffset", "SetSyncDeadTime", "SetBinning", "SetHistoOffset", "SetHistoLen", "SetStopOvl", "SetBitShift", "SetHistoAcqTime", "GetRates", "GetAllRates", "StartMeas", "StopMeas", "AbortMeas", "GetResolution", "GetHistos", "GetAllHistos", "ReadFiFo", "WriteStatus", "Resize", "EnableControls", "DisableControls", "Error", "Exit"]
        # "100 x 60 x 60 x 1000 = 100 h"
        # "Init all FP controls and corresponding copy in UIThread Data cluster"
        # "EnQ list of commands"
        # "Array with Inp.Chan."
        # "Initialization: 1. Init HW -> get # of channels -> make array for Inp.Channels\n2. Init all FP controls and corresponding fields in UIThread Data cluster\n3. EnQ list of commands for further initialization"
        n139 = disable-structure shown="TARGET_TYPE==Windows, Default" {
          disable-tunnel: ["MHLib64" ("name or relative path") "MHLib" ("name or relative path")] -> w316
          frame condition #0 (active) {
          }
          frame condition #1 {
          }
        }
        n140 = xnode "Error Ring"() -> ("error out"=w320:errorcluster)
        n141 = call "GetDLLPath.vi"("DllName_32bit"="MHLib" ("name or relative path"), "DllName_64bit"=w316) -> ("file exists?"=w322:bool, "DLLPath"=w323:path)  [unwired: 8 in]
        n142 = global write "MH_DllPath_global.vi" "DllPath"(w323) -> ()
        n143 = property on="AllChannels" class="Clust (strict)"("Val(Sgnl)"=T1 {"Enable"=TRUE, "Offset"=0, "Level"=-100, "Edge"=0, "DeadTime"=1000, "UseDeadTime"=FALSE, "SetEnableAllChan"=TRUE, "SetEdgeAllChan"=TRUE, "SetLevelAllChan"=TRUE, "SetOffsetAllChan"=TRUE, "SetUseDTAllChan"=TRUE, "SetDeadTAllChan"=TRUE} ("AllChannels")) -> ()  [unwired: 2 in, 2 out]
        n144 = Select(t=errorcluster {"status"=FALSE, "code"=0, "source"=""} ("error IO"), s=w322, f=w320) -> (s? t:f=w337:errorcluster)
        n145 = global read "MH_LibVersion_global.vi" "Library Version"() -> (w318:string)
        n146 = Build Array (concatenate)(w357, w356) -> (w355:T13[])
        n147 = call "InitMH_UIThread.vi"("error in (no error)"=w337, "Mode"=w317, "refsource"=w319, "Library Version"=w318) -> ("error out"=w358:errorcluster, "Init Info"=w360:T10, "DevIdx"=w359:i32)  [unwired: 5 in]
        n148 = local write "SyncDivider"(w354) -> ()
        n149 = local write "SyncOffset"(w353) -> ()
        n150 = local write "SyncEdge"(w352) -> ()
        n151 = local write "SyncLevel"(w351) -> ()
        n152 = local write "Binning"(w350) -> ()
        n153 = Bundle By Name(cluster=w341, "DevIdx"=w359, "Init Info"=w360, "Status"="Initialized!") -> (w340:T9)
        n154 = Unbundle By Name(w340) -> ("Init Info.Bin Steps"=w339:i32, "Init Info.Base Resolution"=w308:dbl, "Init Info.nchannels"=w313:i32)
        n155 = for {
          N: w313 -> [_]
          i -> [w368]
          n156 = Increment(x=w368) -> (x+1=w371:i32)
          n157 = Format Into String(format string="Ch.%d", w371) -> (resulting string=w369:string)  [unwired: 2 in, 1 out]
          n158 = property on="HistoGraph" class="WFGraph (strict)"("Active Plot"=w368, "Plot.Plot Name"=w369) -> ()  [unwired: 2 in, 2 out]
          n159 = property on="TTraceGraph" class="WFGraph (strict)"("Active Plot"=w368, "Plot.Plot Name"=w369) -> ()  [unwired: 2 in, 2 out]
        }
        n160 = Bundle By Name(cluster=T6 {"Histos"=[], "Cmd"=enum."_none_", "TimeTrace"=[], "Bin"=0, "Total bin"=0, "Status"="", "Resol"=0.0, "DeltaT"=0.0, "nChannels"=0} ("MH_GUIThread_QData"), "Cmd"=MH_VisThread_QCmds."nChannels", "nChannels"=w313) -> (w329:T6)
        n161 = To Unsigned Long Integer(number=w308) -> (unsigned 32bit integer=w309:u32)
        n162 = property on="Offset" class="DigNum (strict)"("Increment"=w308) -> ()  [unwired: 2 in, 2 out]
        n163 = property on="SyncOffset" class="DigNum (strict)"("Increment"=w308) -> ()  [unwired: 2 in, 2 out]
        n164 = property on="Offset" class="DigNum (strict)"("Increment"=w308) -> ()  [unwired: 2 in, 2 out]
        n165 = Bundle By Name(cluster=T8 {"Cmd"=enum."Proc", "nActual"=0, "Buffer"=[], "TickCount"=0, "Param"=0} ("MH_DataProcThread_QData"), "Param"=w313, "Cmd"=MH_DataProcThread_QCmds."SetNumChannels") -> (w333:T8)
        n166 = call "MH_CalcBinningValues.vi"("BaseResolution"=w309, "Bin Steps"=w339) -> ("BinningValues"=w344:cluster{"String":string, "Value":i32}[])  [unwired: 9 in]
        n167 = Enqueue Element(queue=w327, element=w329) -> ()  [unwired: 2 in, 3 out]
        n168 = property on="Binning" class="Ring (strict)"("StringsAndValues[]"=w344) -> ()  [unwired: 2 in, 2 out]
        n169 = Enqueue Element(queue=w334, element=w333) -> ()  [unwired: 2 in, 3 out]
        n170 = call "MH_InitChannels.vi"("nchannels"=w313) -> ("SetInpChan"=w311:T11[], "Channels"=w312:T3[])  [unwired: 9 in]
        n171 = local write "Channels"(w312) -> ()
        n172 = Bundle By Name(cluster=w340, "Channels"=w312, "SetInpChan"=w311, "SyncDivider"=w354, "SyncOffset"=w353, "SyncEdge"=w352, "SyncLevel"=w351, "Binning"=w350, "HistoOffset"=w349, "AcqTime"=w348, "StopOvl."=w347, "OvlLevel"=w346, "StartMeas"=w345, "Run cont."=w343, "BitShift"=w326, "HistoAcqTime"=w325, "UseDeadTime"=w315, "SyncDeadTime"=w314) -> (w336:T9)
        n173 = local write "StopOvl."(w347) -> ()
        n174 = local write "OvlLevel"(w346) -> ()
        n175 = local write "Start"(w345) -> ()
        n176 = local write "Run continuously"(w343) -> ()
        n177 = local write "BitShift"(w326) -> ()
        n178 = local write "HistoOffset"(w349) -> ()
        n179 = local write "AcqTime"(w348) -> ()
        n180 = local write "HistoAcqTime"(w325) -> ()
        n181 = local write "UseDeadTime"(w315) -> ()
        n182 = local write "SyncDeadTime"(w314) -> ()
        n183 = property on="Settings" class="Bool (strict)"("Val(Sgnl)"=TRUE ("Value (Signaling)")) -> ()  [unwired: 2 in, 2 out]
        n184 = property on="Scale" class="Bool (strict)"("Val(Sgnl)"=FALSE ("Value (Signaling)")) -> ()  [unwired: 2 in, 2 out]
      }
      frame "SetInpChan" {
        n185 = Unbundle By Name(w379) -> ("DevIdx"=w377:i32, "Init Info.features"=w376:i32, "SetInpChan"=w375:T11[], "Channels"=w374:T3[])
        n186 = for {
          tunnel: w374 -> [w384]
          tunnel: w375 -> [w388] mode=indexing
          shift-right: [w386] -> w373
          shift-left: errorcluster {"status"=FALSE, "code"=0, "source"=""} ("error out") -> [w385]
          tunnel: w377 -> [w382]
          tunnel: w376 -> [w380]
          n187 = Unbundle By Name(w388) -> ("Cmds"=w387:T12[], "Channel"=w381:i32)
          n188 = Index Array(array=w384, index=w381) -> (element=w383:T3)
          n189 = for {
            tunnel: w387 -> [w395] mode=indexing
            tunnel: w381 -> [w394]
            shift-right: [w393] -> w386
            shift-left: w385 -> [w392]
            tunnel: w383 -> [w391]
            tunnel: w382 -> [w390]
            tunnel: w380 -> [w389]
            n190 = case shown="\"SetInpChanDeadTime\"" w395 {
              tunnel: w394 -> [_ w401 w408 w413 w429]
              tunnel: [w396 w400 w407 w417 w434] -> w393
              tunnel: w392 -> [w396 w399 w406 w416 w433]
              tunnel: w391 -> [_ w398 w405 w415 w432]
              tunnel: w390 -> [_ w397 w404 w414 w431]
              tunnel: w389 -> [_ _ _ w410 _]
              frame Default {
              }
              frame "SetInpChanEnable" {
                n191 = Unbundle By Name(w398) -> ("Enable"=w402:bool)
                n192 = call "MH_SetInputChannelEnable.vi"("error in (no error)"=w399, "enable"=w402, "channel"=w401, "devidx"=w397) -> ("error out"=w400:errorcluster)  [unwired: 6 in, 1 out]
              }
              frame "SetInpChanOffset" {
                n193 = Unbundle By Name(w405) -> ("Offset"=w403:i32)
                n194 = call "MH_SetInputChannelOffset.vi"("error in (no error)"=w406, "Offset"=w403, "channel"=w408, "devidx"=w404) -> ("error out"=w407:errorcluster)  [unwired: 6 in, 1 out]
              }
              frame "SetInpChanDeadTime" {
                w411 = 32  # FEATURE_PROG_TD
                n195 = And(x=w410, y=w411) -> (x .and. y?=w412:i32)
                n196 = Not Equal To 0?(x=w412) -> (x != 0?=w409:bool)
                n197 = case shown="False" w409 {
                  tunnel: [w418 w427] -> w417
                  tunnel: w416 -> [w418 w426]
                  tunnel: w415 -> [_ w425]
                  tunnel: w414 -> [_ w424]
                  tunnel: w413 -> [_ w422]
                  frame False {
                  }
                  frame True {
                    n198 = Unbundle By Name(w425) -> ("UseDeadTime"=w421:bool, "DeadTime"=w423:i32)
                    n199 = Boolean To (0,1)(Boolean=w421) -> (0, 1=w420:i16)
                    n200 = To Long Integer(number=w420) -> (32bit integer=w419:i32)
                    n201 = call "MH_SetInputDeadTime.vi"("channel"=w422, "error in (no error)"=w426, "deadtime"=w423, "on"=w419, "devidx"=w424) -> ("error out"=w427:errorcluster)  [unwired: 5 in, 1 out]
                  }
                }
              }
              frame "SetInpChanTrg" {
                n202 = Unbundle By Name(w432) -> ("Level"=w428:i32, "Edge"=w430:i32)
                n203 = call "MH_SetInputEdgeTrg.vi"("channel"=w429, "error in (no error)"=w433, "edge"=w430, "level"=w428, "devidx"=w431) -> ("error out"=w434:errorcluster)  [unwired: 5 in, 1 out]
              }
            }
          }
        }
      }
      frame "SetSyncDivider" {
        n204 = Unbundle By Name(w442) -> ("DevIdx"=w441:i32, "SyncDivider"=w437:i32)
        n205 = Power Of 2(x=w437) -> (2^x=w436:dbl)
        n206 = To Long Integer(number=w436) -> (32bit integer=w435:i32)
        n207 = call "MH_SetSyncDiv.vi"("SyncDivider"=w435, "devidx"=w441) -> ("error out"=w439:errorcluster)  [unwired: 8 in, 1 out]
        n208 = flat-sequence {
          tunnel: w439 -> [w443]
          tunnel: [w443] -> w438
          frame #0 {
            n209 = Wait (ms)(milliseconds to wait=u32 100) -> ()  [unwired: 1 out]
          }
        }
      }
      frame "SetSyncTrg" {
        n210 = Unbundle By Name(w450) -> ("DevIdx"=w447:i32, "SyncLevel"=w445:i32, "SyncEdge"=w446:i32)
        n211 = call "MH_SetSyncEdgeTrg.vi"("edge"=w446, "level"=w445, "devidx"=w447) -> ("error out"=w448:errorcluster)  [unwired: 7 in, 1 out]
      }
      frame "SetSyncDeadTime" {
        w453 = 32  # FEATURE_PROG_TD
        n212 = Unbundle By Name(w462) -> ("DevIdx"=w459:i32, "UseDeadTime"=w456:bool, "SyncDeadTime"=w458:i32, "Init Info.features"=w452:i32)
        n213 = And(x=w452, y=w453) -> (x .and. y?=w454:i32)
        n214 = Boolean To (0,1)(Boolean=w456) -> (0, 1=w457:i16)
        n215 = Not Equal To 0?(x=w454) -> (x != 0?=w451:bool)
        n216 = To Long Integer(number=w457) -> (32bit integer=w455:i32)
        n217 = case shown="True" w451 {
          tunnel: [_ w466] -> w460
          tunnel: w459 -> [_ w465]
          tunnel: w458 -> [_ w464]
          tunnel: w455 -> [_ w463]
          frame False {
          }
          frame True {
            n218 = call "MH_SetSyncDeadTime.vi"("deadtime"=w464, "on"=w463, "devidx"=w465) -> ("error out"=w466:errorcluster)  [unwired: 7 in, 1 out]
          }
        }
      }
      frame "SetSyncOffset" {
        n219 = Unbundle By Name(w471) -> ("DevIdx"=w469:i32, "SyncOffset"=w468:i32)
        n220 = call "MH_SetSyncChannelOffset.vi"("Offset"=w468, "devidx"=w469) -> ("error out"=w470:errorcluster)  [unwired: 8 in, 1 out]
      }
      frame "SetBinning" {
        # "When binning is changed the new resolution is querried"
        n221 = Unbundle By Name(w478) -> ("DevIdx"=w476:i32, "Binning"=w475:i32)
        n222 = call "MH_SetBinning.vi"("Binning"=w475, "devidx"=w476) -> ("error out"=w477:errorcluster)  [unwired: 8 in, 1 out]
        n223 = Build Array (concatenate)(MH_UIThread_Cmds."GetResolution", w473) -> (w474:T13[])
      }
      frame "SetHistoOffset" {
        n224 = Unbundle By Name(w483) -> ("DevIdx"=w480:i32, "HistoOffset"=w479:i32)
        n225 = call "MH_SetOffset.vi"("Offset"=w479, "devidx"=w480) -> ("error out"=w481:errorcluster)  [unwired: 8 in, 1 out]
      }
      frame "SetStopOvl" {
        n226 = Unbundle By Name(w490) -> ("DevIdx"=w487:i32, "StopOvl."=w486:bool, "OvlLevel"=w485:u32)
        n227 = To Unsigned Long Integer(number=w485) -> (unsigned 32bit integer=w484:u32)
        n228 = call "MH_SetStopOverflow.vi"("stopcount"=w484, "StopOnOverflow"=w486, "devidx"=w487) -> ("error out"=w488:errorcluster)  [unwired: 7 in, 1 out]
      }
      frame "SetBitShift" {
        n229 = Unbundle By Name(w494) -> ("BitShift"=w492:i32, "SyncRate"=w493:i32)
        n230 = Negate(x=w492) -> (-x=w502:i32)
        n231 = Bundle By Name(cluster=T8 {"Cmd"=enum."Proc", "nActual"=0, "Buffer"=[], "TickCount"=0, "Param"=0} ("MH_DataProcThread_QData"), "Param"=w502, "Cmd"=MH_DataProcThread_QCmds."SetShift") -> (w508:T8)
        n232 = To Double Precision Float(number=w492) -> (double precision float=w507:dbl)
        n233 = To Double Precision Float(number=w493) -> (double precision float=w506:dbl)
        n234 = Power Of 2(x=w507) -> (2^x=w505:dbl)
        n235 = Enqueue Element(queue=w495, element=w508) -> ()  [unwired: 2 in, 3 out]
        n236 = Multiply(x=w505, y=1000.0) -> (x*y=w504:dbl)
        n237 = Divide(x=w504, y=w506) -> (x/y=w491:dbl)
        "DeltaT" <- w491
        n238 = Bundle By Name(cluster=T6 {"Histos"=[], "Cmd"=enum."_none_", "TimeTrace"=[], "Bin"=0, "Total bin"=0, "Status"="", "Resol"=0.0, "DeltaT"=0.0, "nChannels"=0} ("MH_GUIThread_QData"), "DeltaT"=w491, "Cmd"=MH_VisThread_QCmds."DeltaT") -> (w503:T6)
        n239 = Enqueue Element(queue=w496, element=w503) -> ()  [unwired: 2 in, 3 out]
      }
      frame "SetHistoAcqTime" {
        n240 = Unbundle By Name(w511) -> ("SyncRate"=w517:i32, "HistoAcqTime"=w510:dbl)
        n241 = To Double Precision Float(number=w517) -> (double precision float=w520:dbl)
        n242 = Multiply(x=w520, y=w510) -> (x*y=w519:dbl)
        n243 = Round To Nearest(number=w519) -> (nearest integer value=w518:dbl)
        n244 = To Long Integer(number=w518) -> (32bit integer=w516:i32)
        n245 = Bundle By Name(cluster=T8 {"Cmd"=enum."Proc", "nActual"=0, "Buffer"=[], "TickCount"=0, "Param"=0} ("MH_DataProcThread_QData"), "Param"=w516, "Cmd"=MH_DataProcThread_QCmds."SetHistAcqTime") -> (w515:T8)
        n246 = Enqueue Element(queue=w512, element=w515) -> ()  [unwired: 2 in, 3 out]
      }
      frame "GetAllRates" {
        # "An alternative to GetRates"
        n247 = Unbundle By Name(w523) -> ("DevIdx"=w531:i32, "Init Info.nchannels"=w538:i32, "StartMeas"=w532:bool, "SyncRateStart"=w526:i32)
        n248 = call "MH_AllocateCntRateBuffer.vi"("NumChan"=w538) -> ("Buffer"=w537:i32[])  [unwired: 10 in]
        n249 = call "MH_GetAllCountRates.vi"("cntrates_buf"=w537, "devidx"=w531) -> ("error out"=w530:errorcluster, "cntrates"=→"CountRates":i32[], "syncrate"=w528:i32)  [unwired: 6 in, 1 out]
        n250 = case shown="True" w532 {
          tunnel: w531 -> [_ w553]
          tunnel: w530 -> [w542 w552]
          tunnel: [w542 w551] -> w529
          tunnel: w528 -> [w541 _]
          tunnel: [w541 w548] -> w527
          tunnel: w526 -> [_ w543]
          tunnel: w525 -> [w540 w547]
          tunnel: [w540 w546] -> w524
          tunnel: w523 -> [w539 w545]
          tunnel: [w539 w544] -> w522
          frame False {
          }
          frame True {
            n251 = call "MH_GetSyncPeriod.vi"("error in (no error)"=w552, "devidx"=w553) -> ("error out"=w551:errorcluster, "period"=w550:dbl)  [unwired: 7 in, 1 out]
            n252 = Reciprocal(x=w550) -> (1/x=w549:dbl)
            n253 = To Long Integer(number=w549) -> (32bit integer=w548:i32)
            n254 = case shown="-1" w543 {
              selector: w543 -> [w554 _ _]
              tunnel: w548 -> [w557 w578 _]
              tunnel: w547 -> [w555 w580 w584]
              tunnel: [w556 w580 w584] -> w546
              tunnel: w545 -> [w561 w579 w583]
              tunnel: [w561 w577 w582] -> w544
              frame Default {
                n255 = Subtract(x=w557, y=w554) -> (x-y=w560:i32)
                n256 = Absolute Value(x=w560) -> (abs(x)=w558:i32)
                n257 = Not Equal To 0?(x=w558) -> (x != 0?=w559:bool)
                n258 = case shown="True" w559 {
                  tunnel: w558 -> [_ w570]
                  tunnel: [w562 w565] -> w556
                  tunnel: w555 -> [w562 w564]
                  tunnel: w554 -> [_ w563]
                  frame False {
                  }
                  frame True {
                    n259 = To Double Precision Float(number=w570) -> (double precision float=w569:dbl)
                    n260 = To Double Precision Float(number=w563) -> (double precision float=w571:dbl)
                    n261 = Divide(x=w569, y=w571) -> (x/y=w568:dbl)
                    n262 = Greater Or Equal?(x=w568, y=0.01) -> (x >= y?=w566:bool)
                    n263 = case shown="False" w566 {
                      tunnel: [w572 w575] -> w565
                      tunnel: w564 -> [w572 w573]
                      frame False {
                      }
                      frame True {
                        w574 = T13[] [enum."StopMeas"] items=["Idle", "Init", "SetInpChan", "SetSyncDivider", "SetSyncTrg", "SetSyncOffset", "SetSyncDeadTime", "SetBinning", "SetHistoOffset", "SetHistoLen", "SetStopOvl", "SetBitShift", "SetHistoAcqTime", "GetRates", "GetAllRates", "StartMeas", "StopMeas", "AbortMeas", "GetResolution", "GetHistos", "GetAllHistos", "ReadFiFo", "WriteStatus", "Resize", "EnableControls", "DisableControls", "Error", "Exit"]
                        n264 = One Button Dialog(message="Warning: Sync Rate has changed!\nTime Trace resolution has been changed accordingly.\nMeasurement is aborted.\n") -> ()  [unwired: 1 in, 1 out]
                        n265 = Build Array (concatenate)(w573, w574) -> (w575:T13[])
                      }
                    }
                  }
                }
              }
              frame -1 {
                n266 = Bundle By Name(cluster=w579, "SyncRateStart"=w578) -> (w577:T9)
              }
              frame -2 {
                n267 = Bundle By Name(cluster=w583, "SyncRateStart"=-1) -> (w582:T9)
              }
            }
          }
        }
        n268 = Bundle By Name(cluster=w522, "SyncRate"=w527) -> (w533:T9)
        n269 = Format Into String(format string="Sync Rate: %d cps\n", w527) -> (resulting string=→"SyncRate":string)  [unwired: 2 in, 1 out]
      }
      frame "GetRates" {
        # "An alternative to GetAllRates"
        n270 = Unbundle By Name(w589) -> ("Init Info.nchannels"=w594:i32, "Channels"=w590:T3[], "DevIdx"=w591:i32)
        n271 = call "MH_GetSyncRate.vi"("devidx"=w591) -> ("error out"=w593:errorcluster, "syncrate"=w587:i32)  [unwired: 8 in, 1 out]
        n272 = Format Into String(format string="Sync Rate: %d cps\n", w587) -> (resulting string=w586:string)  [unwired: 2 in, 1 out]
        n273 = local write "SyncRate"(w586) -> ()
        n274 = for {
          N: w594 -> [_]
          tunnel: w591 -> [w602]
          tunnel: [w599] -> w585 mode=indexing
          shift-right: [w601] -> w595
          shift-left: w593 -> [w603]
          tunnel: w590 -> [w598] mode=indexing
          i -> [w600]
          n275 = Unbundle By Name(w598) -> ("Enable"=w597:bool)
          n276 = case shown="True" w597 {
            tunnel: w603 -> [w604 w609]
            tunnel: w602 -> [_ w608]
            tunnel: [w604 w607] -> w601
            tunnel: w600 -> [_ w606]
            tunnel: [_ w605] -> w599
            frame False {
            }
            frame True {
              n277 = call "MH_GetCountRate.vi"("error in (no error)"=w609, "Channel"=w606, "devidx"=w608) -> ("error out"=w607:errorcluster, "rate"=w605:i32)  [unwired: 6 in, 1 out]
            }
          }
        }
        n278 = local write "CountRates"(w585) -> ()
        n279 = Bundle By Name(cluster=w589, "SyncRate"=w587) -> (w588:T9)
      }
      frame "StartMeas" {
        n280 = Bundle By Name(cluster=T8 {"Cmd"=enum."Proc", "nActual"=0, "Buffer"=[], "TickCount"=0, "Param"=0} ("MH_DataProcThread_QData"), "Cmd"=MH_DataProcThread_QCmds."Init") -> (w614:T8)
        n281 = Unbundle By Name(w612) -> ("DevIdx"=w621:i32, "AcqTime"=w617:i32)
        n282 = Enqueue Element(queue=w616, element=w614) -> ()  [unwired: 2 in, 3 out]
        n283 = Bundle By Name(cluster=w612, "SyncRateStart"=-2) -> (w611:T9)
        n284 = call "MH_StartMeas.vi"("tacq"=w617, "devidx"=w621) -> ("error out"=w622:errorcluster)  [unwired: 8 in, 1 out]
        n285 = Build Array (concatenate)(w620, MH_UIThread_Cmds."ReadFiFo") -> (w619:T13[])
      }
      frame "StopMeas" {
        n286 = Unbundle By Name(w628) -> ("Run cont."=w623:bool, "DevIdx"=w629:i32)
        n287 = call "MH_StopMeas.vi"("devidx"=w629) -> ("error out"=w630:errorcluster)  [unwired: 9 in, 1 out]
        n288 = case shown="False" w623 {
          tunnel: w628 -> [w634 w636]
          tunnel: [w633 w636] -> w627
          tunnel: [w631 w635] -> w626
          frame False {
            w631 = T13[] [enum."ReadFiFo"] items=["Idle", "Init", "SetInpChan", "SetSyncDivider", "SetSyncTrg", "SetSyncOffset", "SetSyncDeadTime", "SetBinning", "SetHistoOffset", "SetHistoLen", "SetStopOvl", "SetBitShift", "SetHistoAcqTime", "GetRates", "GetAllRates", "StartMeas", "StopMeas", "AbortMeas", "GetResolution", "GetHistos", "GetAllHistos", "ReadFiFo", "WriteStatus", "Resize", "EnableControls", "DisableControls", "Error", "Exit"]
            w632 = FALSE ("StartMeas")
            n289 = Bundle By Name(cluster=w634, "StartMeas"=w632) -> (w633:T9)
            n290 = local write "Start"(w632) -> ()
          }
          frame True {
            w635 = T13[] [enum."ReadFiFo", enum."StartMeas"] items=["Idle", "Init", "SetInpChan", "SetSyncDivider", "SetSyncTrg", "SetSyncOffset", "SetSyncDeadTime", "SetBinning", "SetHistoOffset", "SetHistoLen", "SetStopOvl", "SetBitShift", "SetHistoAcqTime", "GetRates", "GetAllRates", "StartMeas", "StopMeas", "AbortMeas", "GetResolution", "GetHistos", "GetAllHistos", "ReadFiFo", "WriteStatus", "Resize", "EnableControls", "DisableControls", "Error", "Exit"]
          }
        }
        n291 = Build Array (concatenate)(w625, w626) -> (w624:T13[])
      }
      frame "AbortMeas" {
        w638 = FALSE ("StartMeas")
        n292 = Unbundle By Name(w640) -> ("DevIdx"=w641:i32)
        n293 = call "MH_StopMeas.vi"("devidx"=w641) -> ("error out"=w642:errorcluster)  [unwired: 9 in, 1 out]
        n294 = Bundle By Name(cluster=w640, "StartMeas"=w638) -> (w639:T9)
        n295 = local write "Start"(w638) -> ()
      }
      frame "GetResolution" {
        # "Resolution in ns"
        # "Gets resolution in ps"
        # "Resolution is saved in UIThread Data cluster in ns"
        n296 = Unbundle By Name(w651) -> ("DevIdx"=w653:i32)
        n297 = call "MH_GetResolution.vi"("devidx"=w653) -> ("error out"=w652:errorcluster, "resolution"=w649:dbl)  [unwired: 8 in, 1 out]
        n298 = Divide(x=w649, y=1000.0) -> (x/y=w645:dbl)
        n299 = Bundle By Name(cluster=w651, "Resolution"=w645) -> (w650:T9)
        n300 = Bundle By Name(cluster=T6 {"Histos"=[], "Cmd"=enum."_none_", "TimeTrace"=[], "Bin"=0, "Total bin"=0, "Status"="", "Resol"=0.0, "DeltaT"=0.0, "nChannels"=0} ("MH_GUIThread_QData"), "Resol"=w645, "Cmd"=MH_VisThread_QCmds."Resol") -> (w643:T6)
        n301 = Enqueue Element(queue=w647, element=w643) -> ()  [unwired: 2 in, 3 out]
      }
      frame "ReadFiFo" {
        w663 = 2  # FLAG_FIFOFULL
        # "Reads photon records from HW and transferes them to DataProcThread via Queue."
        n302 = Unbundle By Name(w665) -> ("DevIdx"=w659:i32)
        n303 = call "MH_GetFlags.vi"("devidx"=w659) -> ("error out"=w661:errorcluster, "flags"=w662:i32)  [unwired: 8 in, 1 out]
        n304 = And(x=w662, y=w663) -> (x .and. y?=w664:i32)
        n305 = Not Equal To 0?(x=w664) -> (x != 0?=w658:bool)
        "OverRun" <- w658
        n306 = case shown="False" w658 {
          tunnel: w661 -> [w675 w678]
          tunnel: [w674 w678] -> w660
          tunnel: w659 -> [w667 _]
          tunnel: w657 -> [w673 _]
          tunnel: w656 -> [w672 _]
          tunnel: [w672 w676] -> w655
          frame False {
            n307 = call "MH_ReadFiFo.vi"("error in (no error)"=w675, "devidx"=w667) -> ("error out"=w674:errorcluster, "nactual"=w666:i32, "buffer"=w670:u32[])  [unwired: 6 in, 1 out]
            n308 = Bundle By Name(cluster=T8 {"Cmd"=enum."Proc", "nActual"=0, "Buffer"=[], "TickCount"=0, "Param"=0} ("MH_DataProcThread_QData"), "Buffer"=w670, "nActual"=w666, "Cmd"=MH_DataProcThread_QCmds."Proc") -> (w668:T8)
            n309 = Enqueue Element(queue=w673, element=w668) -> ()  [unwired: 2 in, 3 out]
          }
          frame True {
            n310 = Build Array(MH_UIThread_Cmds."AbortMeas") -> (w676:T13[])
          }
        }
      }
      frame "WriteStatus" {
        n311 = Unbundle By Name(w680) -> ("Status"=→"Status":string)
      }
      frame "Resize" {
        n312 = property on="Pane 3" class="Pane"() -> ("Width"=w687:u32)  [unwired: 2 in, 2 out]
        n313 = Subtract(x=w687, y=i16 100 ("b")) -> (x-y=w693:u32)
        n314 = Unbundle By Name(w682) -> ("Init Info.nchannels"=w690:i32)
        n315 = Quotient & Remainder(x=w693, y=i16 99 ("m")) -> (floor(x/y)=w692:u32)  [unwired: 1 out]
        n316 = In Range and Coerce(upper limit=w690, x=w692, lower limit=4) -> (coerced(x)=w691:u32)  [unwired: 1 out]
        n317 = Equal?(x=w690, y=w691) -> (x = y?=w689:bool)
        n318 = Not(x=w689) -> (.not. x?=w688:bool)
        n319 = property on="Channels" class="Arr (strict)"("HorizScroll"=w688, "Number of Columns"=w691, "Index Values"=u32[] [0]) -> ()  [unwired: 2 in, 2 out]
      }
      frame "EnableControls" {
        n320 = property class="VI"() -> ("Panel"=w698:refnum<vi>)  [unwired: 2 in, 2 out]
        n321 = property class="Pnl"(reference=w698) -> ("Controls[]"=w697:refnum<vi>[])  [unwired: 1 in, 2 out]
        n322 = property class="Pnl"(reference=w698) -> ("Decos[]"=w699:refnum<vi>[])  [unwired: 1 in, 2 out]
        n323 = for {
          tunnel: w699 -> [w703] mode=indexing
          tunnel: TRUE -> [w702]
          n324 = property class="Decor"(reference=w703, "Visible"=w702) -> ()  [unwired: 1 in, 2 out]
        }
        n325 = for {
          tunnel: w697 -> [w706] mode=indexing
          tunnel: T14."Enabled" ("Disabled") -> [w705]
          tunnel: [w704] -> _
          n326 = property class="Ctl"(reference=w706, "DisabledEnum"=w705) -> (error out=w704:errorcluster)  [unwired: 1 in, 1 out]
        }
      }
      frame "DisableControls" {
        n327 = property class="VI"() -> ("Panel"=w710:refnum<vi>)  [unwired: 2 in, 2 out]
        n328 = property class="Pnl"(reference=w710) -> ("Controls[]"=w709:refnum<vi>[])  [unwired: 1 in, 2 out]
        n329 = property class="Pnl"(reference=w710) -> ("Decos[]"=w711:refnum<vi>[])  [unwired: 1 in, 2 out]
        n330 = for {
          tunnel: w711 -> [w715] mode=indexing
          tunnel: FALSE -> [w714]
          n331 = property class="Decor"(reference=w715, "Visible"=w714) -> ()  [unwired: 1 in, 2 out]
        }
        n332 = for {
          tunnel: w709 -> [w718] mode=indexing
          tunnel: T14."Disabled and Grayed Out" ("Disabled") -> [w717]
          tunnel: [w716] -> _
          n333 = property class="Ctl"(reference=w718, "DisabledEnum"=w717) -> (error out=w716:errorcluster)  [unwired: 1 in, 1 out]
        }
      }
      frame "Error" {
        w719 = T13[] [enum."Exit"] items=["Idle", "Init", "SetInpChan", "SetSyncDivider", "SetSyncTrg", "SetSyncOffset", "SetSyncDeadTime", "SetBinning", "SetHistoOffset", "SetHistoLen", "SetStopOvl", "SetBitShift", "SetHistoAcqTime", "GetRates", "GetAllRates", "StartMeas", "StopMeas", "AbortMeas", "GetResolution", "GetHistos", "GetAllHistos", "ReadFiFo", "WriteStatus", "Resize", "EnableControls", "DisableControls", "Error", "Exit"]
        w722 = T18 1 items=["no dialog", "OK message", "continue or stop message", "OK message + warnings", "continue/stop + warnings"] ("type of dialog (OK msg:1)")
        # "Error case: If an error occures the user is informed and the programm terminates. Add your own code to handle error events (e.g. exception lists, etc.)"
        n334 = call <vilib>:"Simple Error Handler.vi"("type of dialog (OK msg:1)"=w722, "error in (no error)"=w721) -> ()  [unwired: 3 in, 5 out]
      }
      frame "Exit" {
        n335 = Release Queue(queue=w724) -> ()  [unwired: 2 in, 3 out]
        n336 = Release Queue(queue=w723) -> ()  [unwired: 2 in, 3 out]
        n337 = Unbundle By Name(w728) -> ("DevIdx"=w727:i32)
        n338 = call "MH_CloseDevice.vi"("devidx"=w727) -> ("error out"=w726:errorcluster)  [unwired: 9 in, 1 out]
      }
    }
    n339 = call "MH_EnQError.vi"("error in (no error)"=w24, "Cmds_in"=w22) -> ("error out"=w23:errorcluster, "Cmds_out"=w21:T13[])  [unwired: 8 in]
  }
  n340 = call "MH_DataProcThread.vi"("MH_VisThread_QRef"=w7, "MH_DataProcThread_QRef"=w1) -> ()  [unwired: 10 in]
  n341 = while {
    tunnel: w7 -> [w737]
    shift-right: [w733] -> _
    shift-left: T5 {"Resol"=0.0, "DeltaT"=0.0, "NumChannels"=0} -> [w734]
    tunnel: w1 -> [w732]
    stop <- w730 stop-if-true
    # "VisualizationThread"
    n342 = Dequeue Element(queue=w737, timeout in ms (-1)=100) -> (element=w735:T6, error out=w730:errorcluster)  [unwired: 1 in, 2 out]
    n343 = Unbundle By Name(w735) -> ("Cmd"=w736:T7)
    n344 = case shown="\"TTrace\"" w736 {
      tunnel: w735 -> [_ w750 w752 w764 w772 w776 w780]
      tunnel: w734 -> [w740 w748 w754 w756 w771 w775 w779]
      tunnel: [w740 w748 w753 w756 w771 w774 w778] -> w733
      tunnel: w732 -> [w739 _ _ _ w768 _ _]
      tunnel: w730 -> [w738 _ _ _ _ _ _]
      frame "_none_", Default {
        n345 = case shown="No Error" w738 {
          tunnel: w739 -> [w744 _]
          frame No Error {
            n346 = Get Queue Status(queue=w744) -> (# elements in queue=w742:i32)  [unwired: 2 in, 7 out]
            n347 = Format Into String(format string="Elements in Q: %d", w742) -> (resulting string=w741:string)  [unwired: 2 in, 1 out]
            n348 = local write "Status"(w741) -> ()
          }
          frame Error {
          }
        }
      }
      frame "Histo" {
        n349 = Unbundle By Name(w750) -> ("Histos"=w745:u32[][])
        n350 = Unbundle By Name(w748) -> ("Resol"=w747:dbl)
        n351 = Bundle(0.0, "Resol"=w747, "Histos"=w745) -> (→"HistoGraph":cluster{dbl, "Resol":dbl, "Histos":u32[][]})  [unwired: 1 in]
      }
      frame "nChannels" {
        n352 = Unbundle By Name(w752) -> ("nChannels"=w751:i32)
        n353 = Bundle By Name(cluster=w754, "NumChannels"=w751) -> (w753:T5)
      }
      frame "TTrace" {
        n354 = Unbundle By Name(w764) -> ("Total bin"=w763:u64, "Bin"=w762:i32, "TimeTrace"=w761:u32[][])
        n355 = Unbundle By Name(w756) -> ("DeltaT"=w755:dbl)
        n356 = call "MH_TTraceToGraph.vi"("DeltaT"=w755, "TimeTrace"=w761, "Bin"=w762, "Total bin"=w763) -> ("TimeTrace_out"=w758:u32[][], "dt"=w759:dbl, "T0"=w760:dbl)  [unwired: 5 in]
        n357 = Bundle("T0"=w760, "dt"=w759, "TimeTrace_out"=w758) -> (→"TTraceGraph":T19)  [unwired: 1 in]
      }
      frame "Status" {
        n358 = Unbundle By Name(w772) -> ("Status"=w769:string)
        n359 = Get Queue Status(queue=w768) -> (# elements in queue=w767:i32)  [unwired: 2 in, 7 out]
        n360 = Format Into String(format string="\t\tElements in Q: %d", w767) -> (resulting string=w765:string)  [unwired: 2 in, 1 out]
        n361 = Concatenate Strings(w769, w765) -> (w770:string)
        n362 = local write "Status"(w770) -> ()
      }
      frame "DeltaT" {
        n363 = Unbundle By Name(w776) -> ("DeltaT"=w773:dbl)
        n364 = Bundle By Name(cluster=w775, "DeltaT"=w773) -> (w774:T5)
      }
      frame "Resol" {
        n365 = Unbundle By Name(w780) -> ("Resol"=w777:dbl)
        n366 = Bundle By Name(cluster=w779, "Resol"=w777) -> (w778:T5)
      }
    }
  }
